vi "write_data_with_UDP.vi"(5 "port":u16, 7 "address":u32, 8 "error_in":errorcluster, 10 "data_in":dbl[](array[numeric]), 11 "udp_ref_in":refnum<k16>) -> (0 "error_out":errorcluster, 3 "udp_ref_out":refnum<k16>)   [LabVIEW 2020]
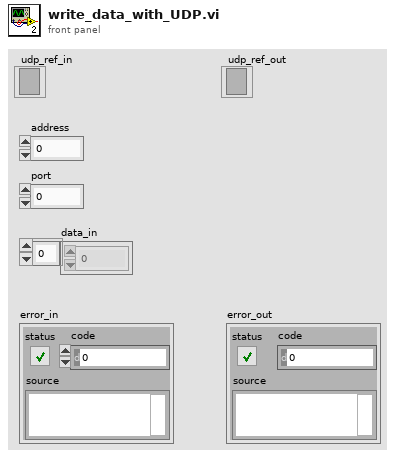
[diagram p1: front panel]
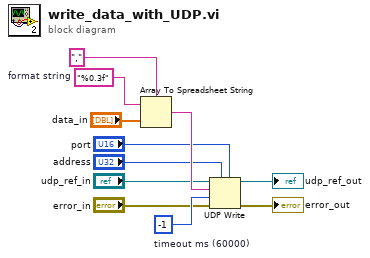
[diagram p0: block diagram]
diagram:
  w10 = -1  # timeout ms (60000)
  w6 = "%0.3f"  # format string
  n1 = Array To Spreadsheet String(delimiter (Tab)=",", array="data_in", 3:w6) -> (spreadsheet string=w11:string)
  n2 = UDP Write(address="address", port or service name="port", connection ID="udp_ref_in", data in=w11, 8:"error_in", 9:w10) -> (error out=→"error_out":errorcluster, 3:→"udp_ref_out":refnum<k16>)
